vi "题目2.vi"() -> ()   [LabVIEW 2017]
panel:
  out "数字波形图":digitalwaveform(graph)
  in  "digital waveform":digitalwaveform(waveform) caption="数字波形"
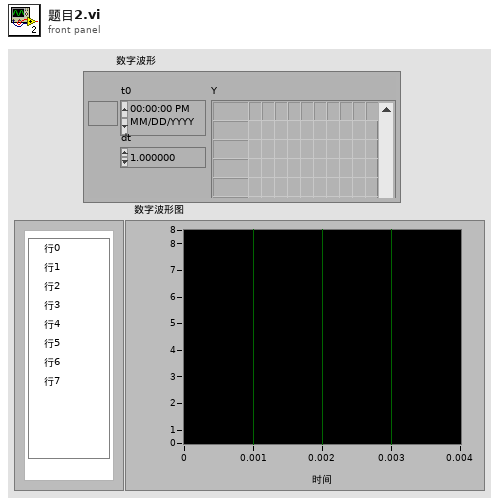
[diagram p1: front panel]
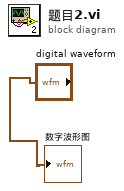
[diagram p0: block diagram]
diagram:
  "数字波形图" <- "digital waveform"
